vi "trafienie.vi"(2 "miny":i32[][](array[numeric]), 3 "rozmiar":i32) -> (1 "Array 2":i32[][](array[numeric]))   [LabVIEW 2016]
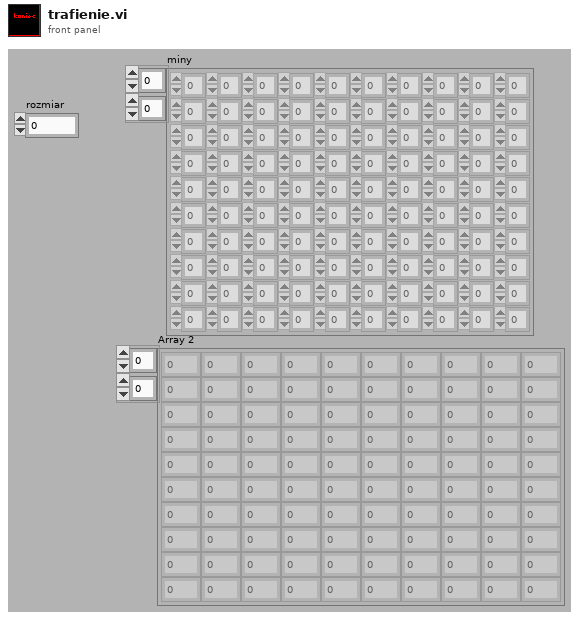
[diagram p1: front panel]
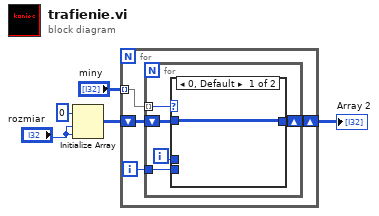
[diagram p0: block diagram]
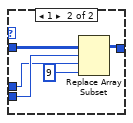
[diagram p2: hidden frame]
diagram:
  n1 = Initialize Array(0 ("element"), "rozmiar", "rozmiar") -> (w5:i32[][])
  n2 = for {
    shift-right: [w8] -> w2
    shift-left: w5 -> [w9]
    tunnel: "miny" -> [w6] mode=indexing
    i -> [w7]
    n3 = for {
      shift-right: [w11] -> w8
      shift-left: w9 -> [w14]
      tunnel: w7 -> [w13]
      tunnel: w6 -> [w10] mode=indexing
      i -> [w12]
      n4 = case shown="0, Default" w10 {
        tunnel: [w15 w19] -> w11
        tunnel: w14 -> [w15 w20]
        tunnel: w13 -> [_ w17]
        tunnel: w12 -> [_ w16]
        frame 0, Default {
        }
        frame 1 {
          n5 = Replace Array Subset(array=w20, new element=9 ("CONTADOR"), index (row)=w17, index (col)=w16) -> (w19:i32[][])
        }
      }
    }
  }
  "Array 2" <- w2
